vi "A13rowin.vi"(0 "Basic Size":dbl, 3 "error in":errorcluster) -> (5 "Row":i32, 8 "error out":errorcluster)   [LabVIEW 2023]
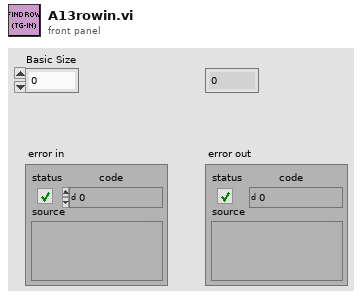
[diagram p1: front panel]
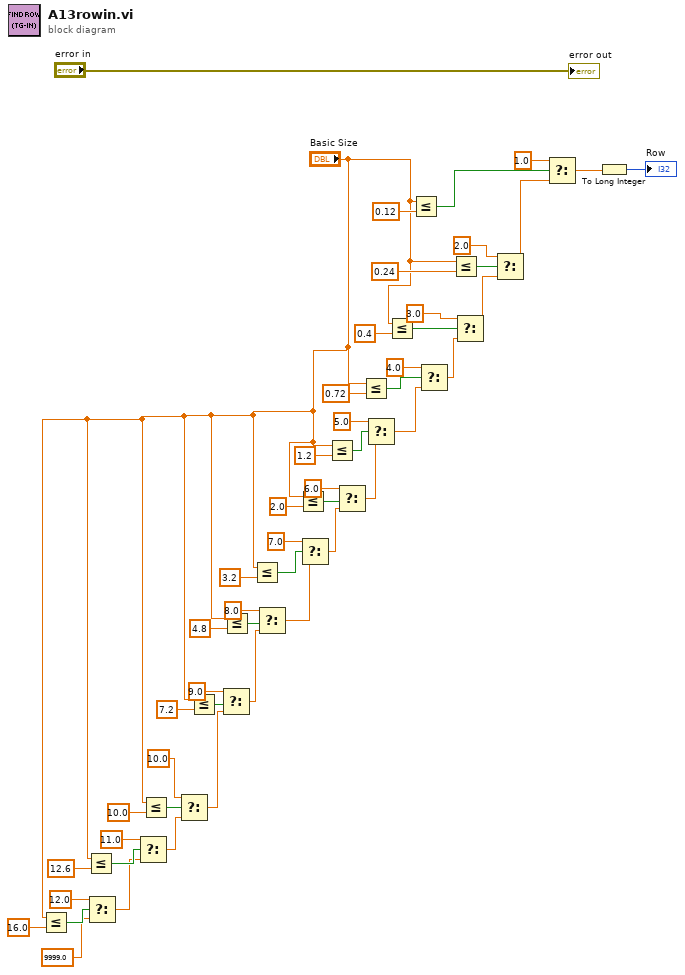
[diagram p0: block diagram]
diagram:
  n1 = Less Or Equal?(x="Basic Size", y=16.0) -> (x <= y?=w7:bool)
  n2 = Less Or Equal?(x="Basic Size", y=12.6) -> (x <= y?=w11:bool)
  n3 = Select(t=12.0, s=w7, f=9999.0) -> (s? t:f=w9:dbl)
  n4 = Select(t=11.0, s=w11, f=w9) -> (s? t:f=w13:dbl)
  n5 = Less Or Equal?(x="Basic Size", y=10.0) -> (x <= y?=w15:bool)
  n6 = Select(t=10.0, s=w15, f=w13) -> (s? t:f=w17:dbl)
  n7 = Less Or Equal?(x="Basic Size", y=7.2) -> (x <= y?=w19:bool)
  n8 = Select(t=9.0, s=w19, f=w17) -> (s? t:f=w21:dbl)
  n9 = Less Or Equal?(x="Basic Size", y=4.8) -> (x <= y?=w23:bool)
  n10 = Less Or Equal?(x="Basic Size", y=3.2) -> (x <= y?=w27:bool)
  n11 = Select(t=8.0, s=w23, f=w21) -> (s? t:f=w25:dbl)
  n12 = Less Or Equal?(x="Basic Size", y=2.0) -> (x <= y?=w31:bool)
  n13 = Select(t=7.0, s=w27, f=w25) -> (s? t:f=w29:dbl)
  n14 = Less Or Equal?(x="Basic Size", y=1.2) -> (x <= y?=w35:bool)
  n15 = Select(t=6.0, s=w31, f=w29) -> (s? t:f=w33:dbl)
  n16 = Less Or Equal?(x="Basic Size", y=0.72) -> (x <= y?=w39:bool)
  n17 = Select(t=5.0, s=w35, f=w33) -> (s? t:f=w37:dbl)
  n18 = Less Or Equal?(x="Basic Size", y=0.4) -> (x <= y?=w43:bool)
  n19 = Less Or Equal?(x="Basic Size", y=0.12) -> (x <= y?=w52:bool)
  n20 = Select(t=4.0, s=w39, f=w37) -> (s? t:f=w41:dbl)
  n21 = Less Or Equal?(x="Basic Size", y=0.24) -> (x <= y?=w48:bool)
  n22 = Select(t=3.0, s=w43, f=w41) -> (s? t:f=w45:dbl)
  n23 = Select(t=2.0, s=w48, f=w45) -> (s? t:f=w50:dbl)
  n24 = Select(t=1.0, s=w52, f=w50) -> (s? t:f=w3:dbl)
  n25 = To Long Integer(number=w3) -> (32bit integer=→"Row":i32)
  "error out" <- "error in"
